vi "Read Bool.vi"(6 "timeout ms (1000)":i32=1000, 7 "Function Code":T1 items=["None"=0, "Read Coil Status"=1, "Read Input Status"=2, "Read Holding Registers"=3, "Read Input Registers"=4, "Force Single Coil"=5, "Preset Single Register"=6, "Force Multiple Coils"=15, "Preset Multiple Registers"=16], 8 "error in (no error)":errorcluster, 9 "Number of Registers":u16, 10 "Start Address":u16, 11 "TCP Network Connection in":refnum<k5>) -> (0 "error out":errorcluster, 2 "Values":bool[](array[boolean]), 3 "TCP Network Connection out":refnum<k5>)   [LabVIEW 2023, in "Modbus TCP Micro.lvlib"]
uses:
  Modbus TCP Micro.lvlib
  Modbus Functions.ctl
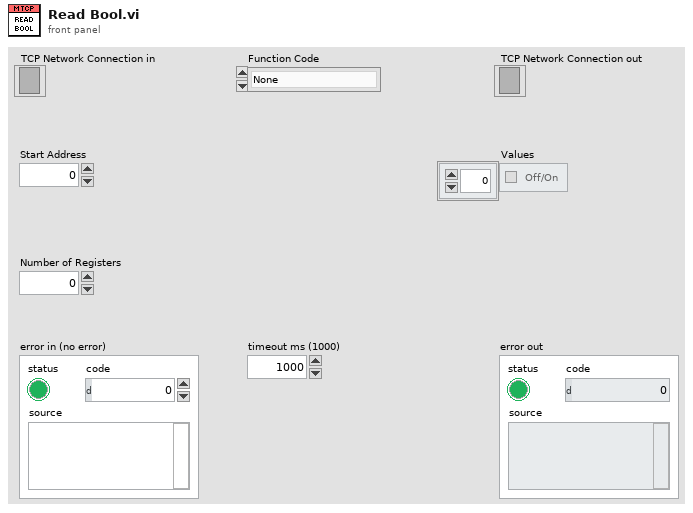
[diagram p1: front panel]
types:
  T1 = typedef "Modbus TCP Micro.lvlib/Modbus Functions.ctl" = u8
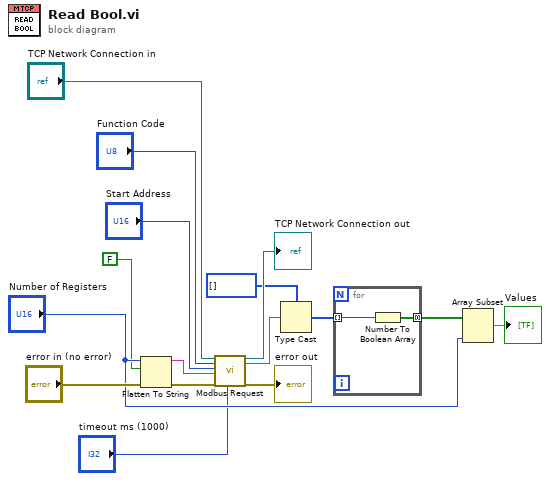
[diagram p0: block diagram]
diagram:
  n1 = Flatten To String(anything="Number of Registers", prepend array or string size? (T)=FALSE, error in (no error)="error in (no error)") -> (data string=w4:string, error out=w7:errorcluster)  [unwired: 1 in, 1 out]
  n2 = call "Modbus Request.vi"("TCP Network Connection in"="TCP Network Connection in", "Function Codes"="Function Code", "Start Address"="Start Address", "Payload"=w4, "error in (no error)"=w7, "timeout ms (1000)"="timeout ms (1000)") -> ("TCP Network Connection out"=→"TCP Network Connection out":refnum<k5>, "Payload"=w9:string, "error out"=→"error out":errorcluster)  [unwired: 8 in, 3 out]
  n3 = Type Cast(type=u8[] [], x=w9) -> (*(type *) &x=w14:u8[])
  n4 = for {
    tunnel: w14 -> [w18] mode=indexing
    tunnel: [w17] -> w15 mode=concatenating
    n5 = Number To Boolean Array(number=w18) -> (Boolean array=w17:bool[])
  }
  n6 = Array Subset(array=w15, length="Number of Registers") -> (→"Values":bool[])  [unwired: 1 in]
